vi "Write remote port.vi"(8 "error in (no error)":errorcluster, 10 "remote port (80)":u16=80, 11 "Connection.TCP":refnum<class "Connection.TCP.lvclass">) -> (0 "error out":errorcluster, 3 "Connection.TCP":refnum<class "Connection.TCP.lvclass">)   [LabVIEW 2013, in "Connection.TCP_GOSPL.lvlib" / "Connection.TCP.lvclass"]
uses:
  Connection.TCP.lvclass
  Connection.TCP.lvclass/Connection.TCP.ctl
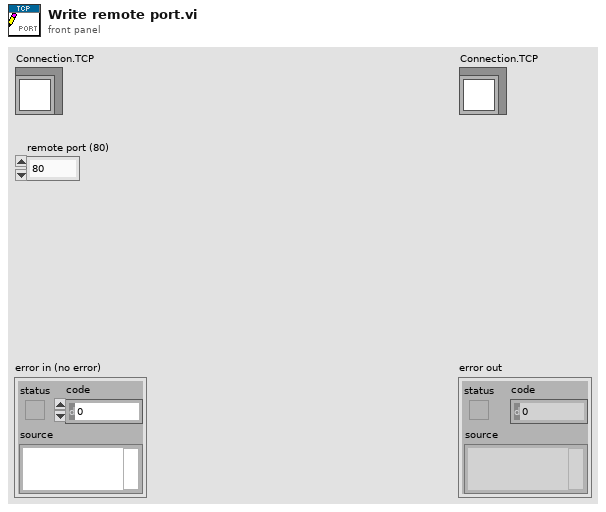
[diagram p1: front panel]
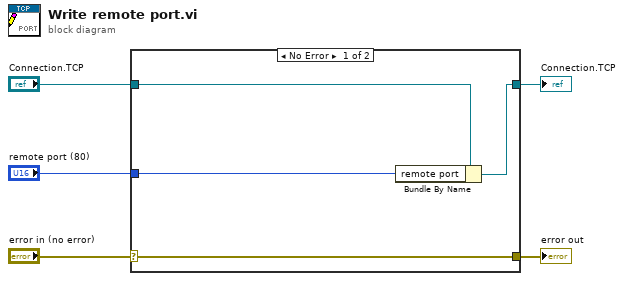
[diagram p0: block diagram]
diagram:
  n1 = case shown="No Error" "error in (no error)" {
    selector: "error in (no error)" -> [w9 w10]
    tunnel: [w9 w10] -> w4
    tunnel: [w7 w11] -> w2
    tunnel: "Connection.TCP" -> [w8 w11]
    tunnel: "remote port (80)" -> [w6 _]
    frame No Error {
      n2 = Bundle By Name(cluster=w8, "remote port"=w6) -> (w7:refnum<class "Connection.TCP.lvclass">)
    }
    frame Error {
    }
  }
  "error out" <- w4
  "Connection.TCP" <- w2
